vi "Main.vi"() -> ()   [LabVIEW 2021]
uses:
  ctrl/5110_trigger.ctl
  ctrl/ini-stop-read.ctl
  ctrl/5110_q.ctl
  ctrl/create-rw-close.ctl
  ctrl/ini-rw.ctl
  ctrl/rw.ctl
  ctrl/5110_cmd.ctl
panel:
  in  "Tab Control":enum32{"User Interface", "Config"}(tab)
  in  "arr size":u16=100
  in  "Color":bool
  out "Intensity Graph":dbl[][](graph)
  in  "Stop":bool
  in  "Exit":bool
  out "Waveform Graph":T1(graph)
  in  "line":i32
  in  "PXI-5110 cfg":T2={"visa"="Dev1", "Channel Name"="0", "Enforce Realtime"=TRUE, "Vertical Range"=5.0, "Min Sample Rate"=10000000.0, "Min Record Length"=1000, "Actual Record Length"=1000, "Actual Sample Rate"=10000000.0, "Timeout (s)"=5.0, "Vertical Offset"=0.0, "Probe Attenuation"=1.0, "Input Impedance"=0, "Maximum Input Frequency"=0.0, "Vertical Coupling"=1, "Trigger"={"Coupling"=1, "Trigger Slope"=0, "Trigger Level"=0.0, "Trigger Source"="0", "Trigger Delay"=0.0, "Reference Position"=50.0, "Trigger Modifier"=2, "Auto Triggered"=FALSE}} {"Trigger"."Trigger Modifier" items=["None"=1, "Auto Trigger"=2]; "Trigger"."Reference Position" format="%.1f"; "Trigger"."Trigger Delay" format="%#.4p"; "Trigger"."Trigger Level" format="%.2f"; "Trigger"."Trigger Slope" items=["Positive", "Negative"]; "Trigger"."Coupling" items=["AC"=0, "DC"=1, "HF Reject"=3, "LF Reject"=4, "AC Plus HF Reject"=1001]; "Vertical Coupling" items=["AC", "DC", "Ground"]; "Maximum Input Frequency" format="%.2f"; "Input Impedance" items=["1 mega ohm"=0, "50 ohms"=2]; "Probe Attenuation" format="%.1f"; "Vertical Offset" format="%.2p"; "Timeout (s)" format="%.2f"; "Actual Sample Rate" format="%#.2p"; "Min Sample Rate" step=1000000.0 format="%#.2p"; "Vertical Range" format="%.2f"}
  in  "Custom Marker Colors":u32[](array[colorbox])=[16714752, 16748562, 16773418]
  # "Vertical"
  # "Channel"
  # "Horizontal"
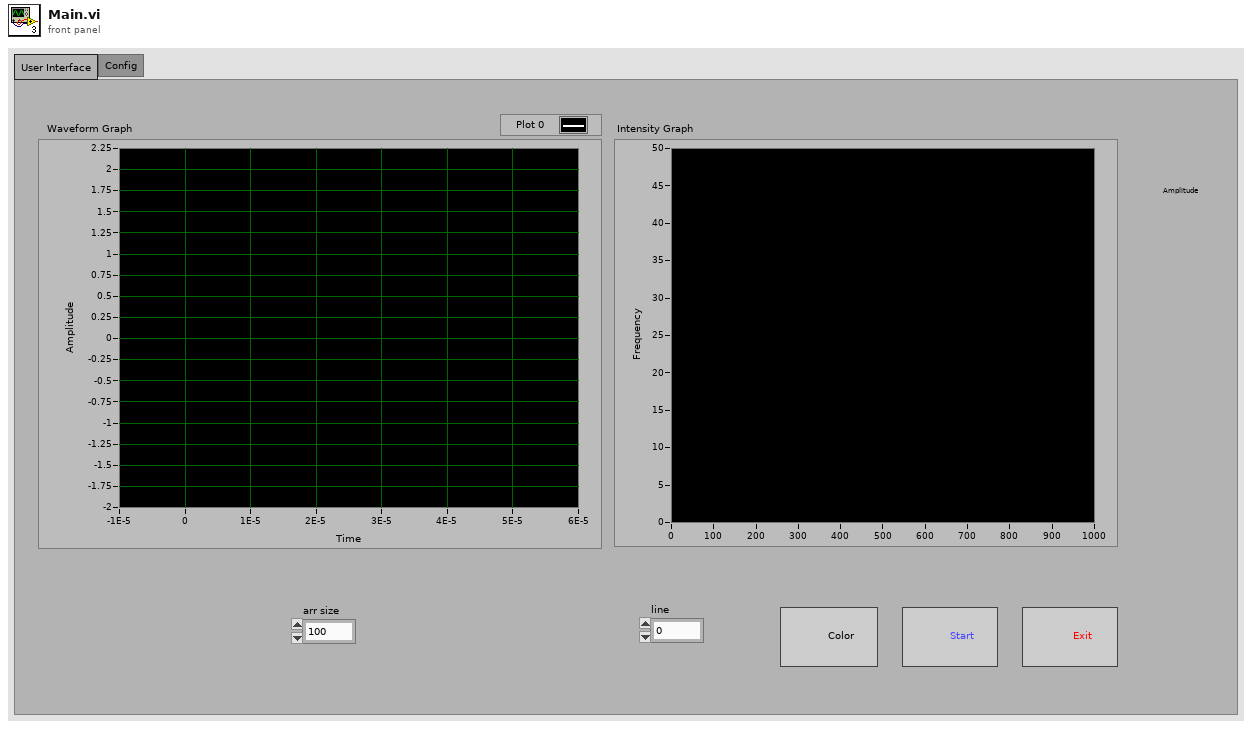
[diagram p1: front panel]
types:
  T1 = cluster{"relativeInitialX":dbl, "xIncrement":dbl, "wfm":dbl[]}
  T2 = typedef "5110_trigger.ctl" = cluster{"visa":refnum<k15>, "Channel Name":string, "Enforce Realtime":bool, "Vertical Range":dbl, "Min Sample Rate":dbl, "Min Record Length":i32, "Actual Record Length":i32, "Actual Sample Rate":dbl, "Timeout (s)":dbl, "Vertical Offset":dbl, "Probe Attenuation":dbl, "Input Impedance":u32, "Maximum Input Frequency":dbl, "Vertical Coupling":i32, "Trigger":cluster{"Coupling":u16, "Trigger Slope":i32, "Trigger Level":dbl, "Trigger Source":string, "Trigger Delay":dbl, "Reference Position":dbl, "Trigger Modifier":i32, "Auto Triggered":bool}}
  T3 = typedef "ini-rw.ctl" = enum16{"read", "write", "ini"}
  T4 = typedef "create-rw-close.ctl" = enum16{"create", "read", "write", "close"}
  T5 = typedef "5110_q.ctl" = enum16{"create", "read", "write", "close"}
  T6 = typedef "ini-stop-read.ctl" = enum16{"init", "stop", "read"}
  T7 = typedef "rw.ctl" = enum16{"read", "write"}
  T8 = typedef "5110_cmd.ctl" = enum16{"check", "run", "stop"}
  T9 = cluster{"Waveform(s)":cluster{"relativeInitialX":dbl, "xIncrement":dbl, "wfm":dbl[]}[], "Actual Record Length":i32, "Actual Sample Rate":dbl, "Auto Triggered":bool}
  T10 = cluster{"relativeInitialX":dbl, "xIncrement":dbl, "wfm":dbl[]}[]
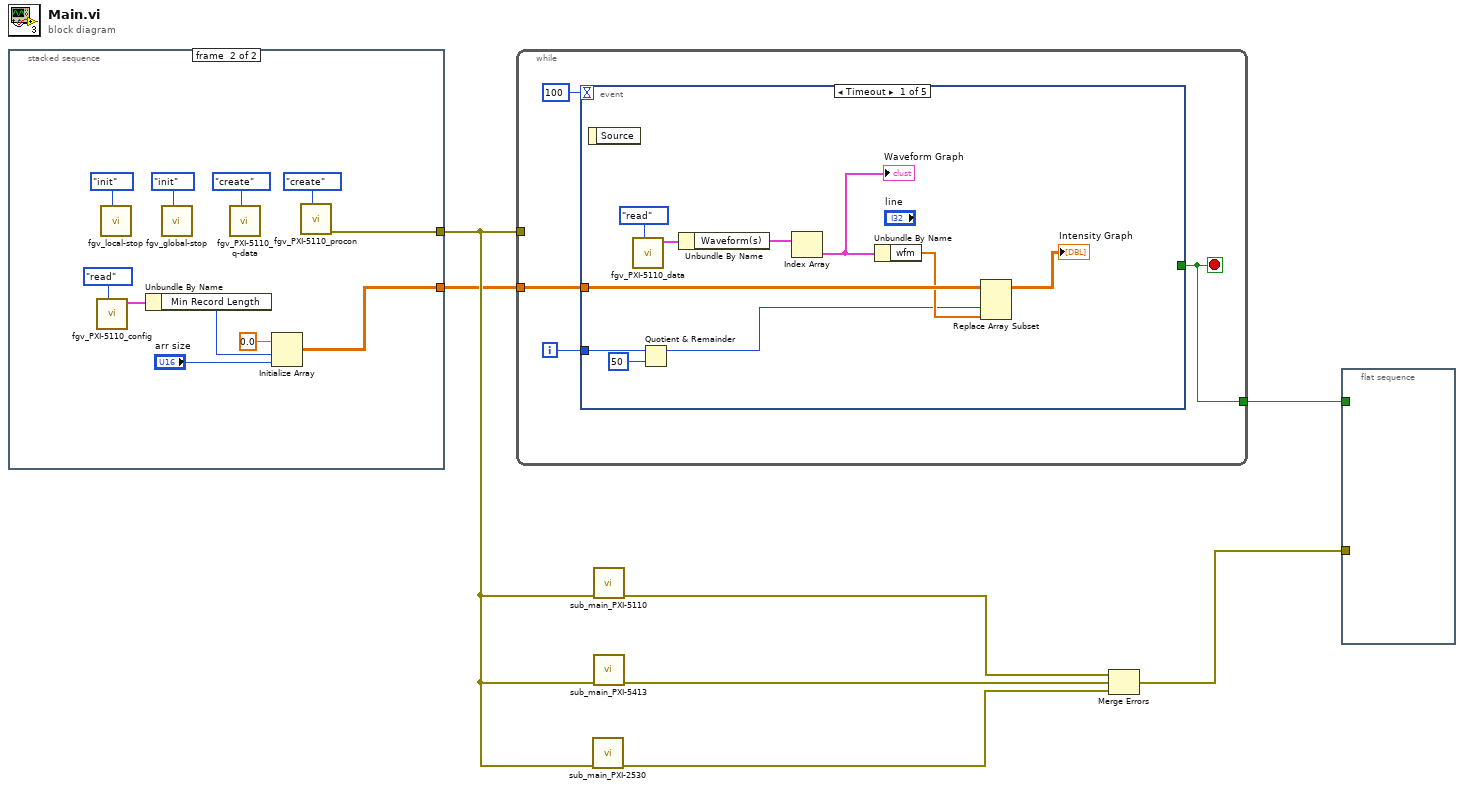
[diagram p0: block diagram]
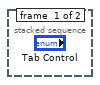
[diagram p2: hidden frame]
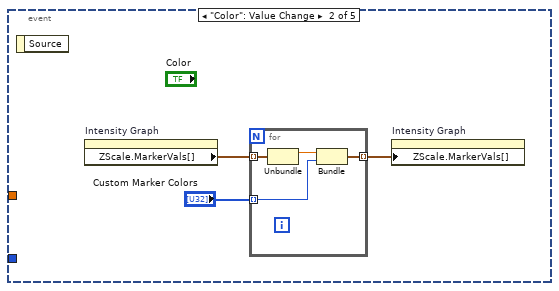
[diagram p3: hidden frame]
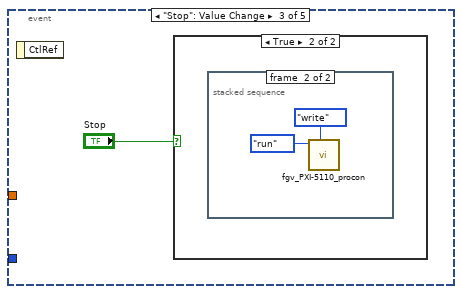
[diagram p4: hidden frame]
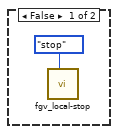
[diagram p5: hidden frame]
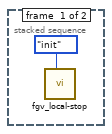
[diagram p6: hidden frame]
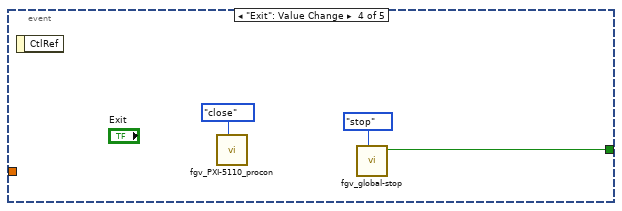
[diagram p7: hidden frame]
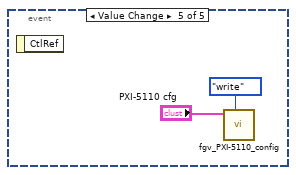
[diagram p8: hidden frame]
diagram:
  n1 = stacked-sequence {
    tunnel: [_ w9] -> w3
    tunnel: [_ w8] -> w1
    frame #0 {
    }
    frame #1 {
      n2 = call "fgv_PXI-5110_config.vi"("cmd"=ini-rw."read") -> ("cfg 2"=w13:T2)  [unwired: 10 in]
      n3 = call "fgv_local-stop.vi"("cmd"=ini-stop-read."init") -> ()  [unwired: 10 in, 1 out]
      n4 = Unbundle By Name(w13) -> ("Min Record Length"=w12:i32)
      n5 = call "fgv_global-stop.vi"("cmd"=ini-stop-read."init") -> ()  [unwired: 10 in, 1 out]
      n6 = call "fgv_PXI-5110_q-data.vi"("cmd"=5110_q."create") -> ()  [unwired: 9 in, 2 out]
      n7 = Initialize Array(0.0, w12, "arr size") -> (w8:dbl[][])
      n8 = call "fgv_PXI-5110_procon.vi"("cmd"=create-rw-close."create") -> ("error out"=w9:errorcluster)  [unwired: 9 in, 1 out]
    }
  }
  n9 = while {
    tunnel: w3 -> [_]
    tunnel: [w21] -> w7
    tunnel: w1 -> [w20]
    i -> [w19]
    stop <- w21 stop-if-true
    n10 = event shown="[0] Timeout" {
      selector: _ -> [_ _ _ _ _]
      dyn-events: _ -> [_ _ _ _ _]
      timeout: 100 -> [_ _ _ _ _]
      tunnel: [_ _ _ w46 _] -> w21
      tunnel: w20 -> [w26 _ _ _ _]
      tunnel: w19 -> [w28 _ _ _ _]
      event Timeout {
        n11 = event-data() -> ()  [unwired: 1 in, 1 out]
        n12 = call "fgv_PXI-5110_data.vi"("cmd"=rw."read") -> ("data 2"=w31:T9)  [unwired: 10 in]
        n13 = Quotient & Remainder(x=w28, y=50) -> (x-y*floor(x/y)=w24:i32)  [unwired: 1 out]
        n14 = Unbundle By Name(w31) -> ("Waveform(s)"=w30:T10)
        n15 = Index Array(array=w30) -> (element=w29:T1)  [unwired: 1 in]
        "Waveform Graph" <- w29
        n16 = Unbundle By Name(w29) -> ("wfm"=w25:dbl[])
        n17 = Replace Array Subset(array=w26, new element=w25, index (col)=w24) -> (→"Intensity Graph":dbl[][])  [unwired: 1 in]
      }
      event "Color": Value Change {
        n18 = event-data() -> ()  [unwired: 1 in, 1 out]
        n19 = property on="Intensity Graph" class="IntensityGraph (strict)"() -> ("ZScale.MarkerVals[]"=w33:cluster{dbl, u32}[])  [unwired: 2 in, 2 out]
        n20 = for {
          tunnel: w33 -> [w39] mode=indexing
          tunnel: "Custom Marker Colors" -> [w37] mode=indexing
          tunnel: [w36] -> w35 mode=indexing
          n21 = Unbundle(w39) -> (w38:dbl)  [unwired: 1 out]
          n22 = Bundle(w38, "Color Box"=w37) -> (w36:cluster{dbl, "Color Box":u32})  [unwired: 1 in]
        }
        n23 = property on="Intensity Graph" class="IntensityGraph (strict)"("ZScale.MarkerVals[]"=w35) -> ()  [unwired: 2 in, 2 out]
      }
      event "Stop": Value Change {
        n24 = event-data() -> ()  [unwired: 1 in, 1 out]
        n25 = case shown="True" "Stop" {
          frame False {
            n26 = call "fgv_local-stop.vi"("cmd"=ini-stop-read."stop") -> ()  [unwired: 10 in, 1 out]
          }
          frame True {
            n27 = stacked-sequence {
              frame #0 {
                n28 = call "fgv_local-stop.vi"("cmd"=ini-stop-read."init") -> ()  [unwired: 10 in, 1 out]
              }
              frame #1 {
                n29 = call "fgv_PXI-5110_procon.vi"("cmd"=create-rw-close."write", "data"=5110_cmd."run") -> ()  [unwired: 8 in, 2 out]
              }
            }
          }
        }
      }
      event "Exit": Value Change {
        n30 = event-data() -> ()  [unwired: 1 in, 1 out]
        n31 = call "fgv_PXI-5110_procon.vi"("cmd"=create-rw-close."close") -> ()  [unwired: 9 in, 2 out]
        n32 = call "fgv_global-stop.vi"("cmd"=ini-stop-read."stop") -> ("stop"=w46:bool)  [unwired: 10 in]
      }
      event Value Change {
        n33 = event-data() -> ()  [unwired: 1 in, 1 out]
        n34 = call "fgv_PXI-5110_config.vi"("cmd"=ini-rw."write", "cfg"="PXI-5110 cfg") -> ()  [unwired: 9 in, 1 out]
      }
    }
  }
  n35 = call "sub_main_PXI-2530.vi"("error in"=w3) -> ("error out"=w2:errorcluster)  [unwired: 10 in]
  n36 = call "sub_main_PXI-5110.vi"("error in"=w3) -> ("error out"=w6:errorcluster)  [unwired: 10 in]
  n37 = call "sub_main_PXI-5413.vi"("error in"=w3) -> ("error out"=w5:errorcluster)  [unwired: 10 in]
  n38 = Merge Errors(w6, w5, w2) -> (w4:errorcluster)
  n39 = flat-sequence {
    tunnel: w7 -> [_]
    tunnel: w4 -> [_]
    frame #0 {
    }
  }
